vi "_093.vi"() -> ()   [LabVIEW 2020]
panel:
  out "x/y":dbl
  in  "stop":bool
  # "What does this vi have a race condition ?"
  # "There is nothing to control the execution of the two local variables."
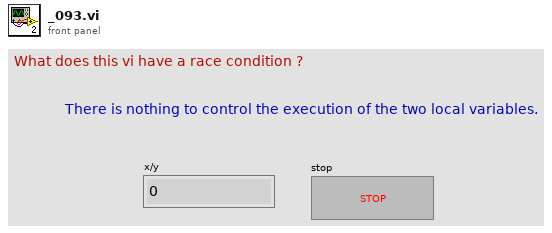
[diagram p1: front panel]
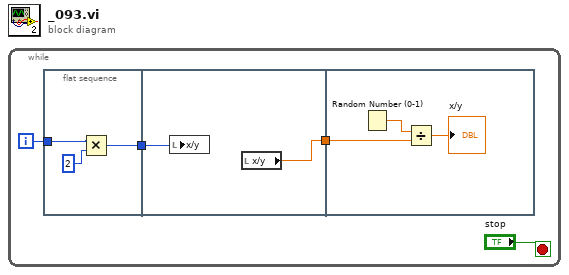
[diagram p0: block diagram]
diagram:
  n1 = while {
    i -> [w3]
    stop <- "stop" stop-if-true
    n2 = flat-sequence {
      tunnel: w3 -> [w6]
      tunnel: [w5] -> w2
      tunnel: w2 -> [w8]
      tunnel: [w9] -> w1
      tunnel: w1 -> [w11]
      frame #0 {
        n3 = Multiply(x=w6, y=2) -> (x*y=w5:i32)
      }
      frame #1 {
        n4 = local write "x/y"(w8) -> ()
        n5 = local read "x/y"() -> (w9:dbl)
      }
      frame #2 {
        n6 = Random Number (0-1)() -> (number: 0 to 1=w12:dbl)
        n7 = Divide(x=w12, y=w11) -> (x/y=→"x/y":dbl)
      }
    }
  }
